vi "Feature extraction.vi"(10 "Utterance Frames":dbl[][](array[numeric])) -> (2 "Acoustic vector":dbl[][](array[numeric]))   [LabVIEW 2013]
uses:
  <vilib>/Analysis/2dsp.llb/Real FFT.vi
  <vilib>/Analysis/2dsp.llb/1D DCT.vi
  <vilib>/Analysis/baseanly.llb/Mean (DBL).vi
  <vilib>/Analysis/NI_AALPro.lvlib
  <vilib>/Analysis/NI_AALBase.lvlib
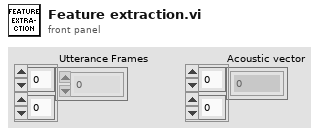
[diagram p1: front panel]
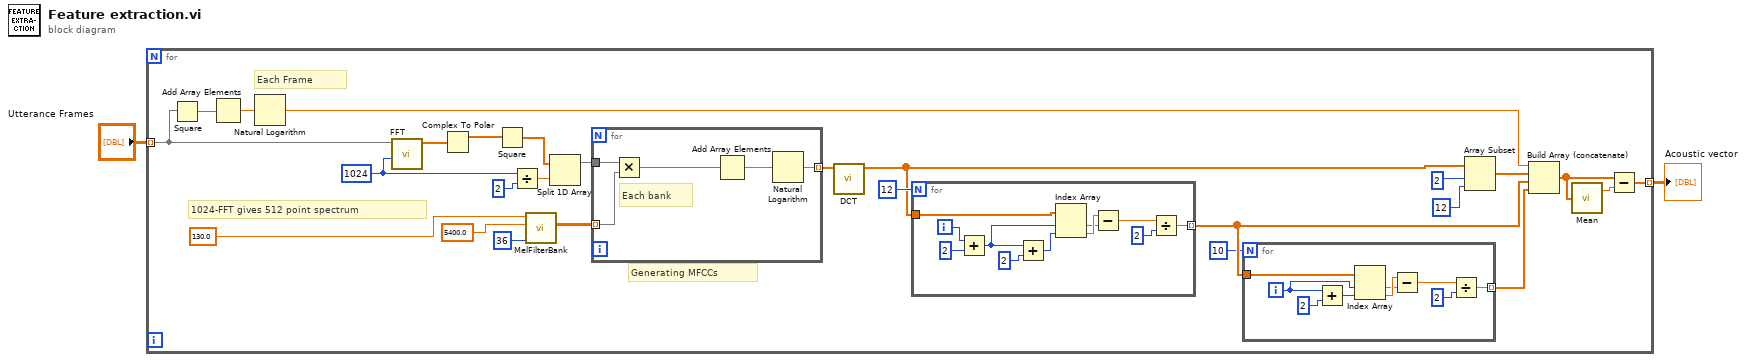
[diagram p0: block diagram]
diagram:
  n1 = for {
    tunnel: "Utterance Frames" -> [w17] mode=indexing
    tunnel: [w3] -> w2 mode=indexing
    w21 = 1024 ("FFT size")
    # "Each Frame"
    # "Generating MFCCs"
    # "1024-FFT gives 512 point spectrum"
    n2 = Square(x=w17) -> (x^2=w16:dbl[])
    n3 = Add Array Elements(numeric array=w16) -> (sum=w15:dbl)
    n4 = Natural Logarithm(1:w15) -> (0:w10:dbl)
    n5 = call-poly <vilib>:"FFT.vi"("FFT size"=w21, "X"=w17) -> ("FFT {X}"=w23:cdb[])  [unwired: 8 in, 1 out]
    n6 = Complex To Polar(r * e^(i*theta)=w23) -> (r=w22:dbl[])  [unwired: 1 out]
    n7 = Square(x=w22) -> (x^2=w18:dbl[])
    n8 = Divide(x=w21, y=2 ("FFT size")) -> (x/y=w19:dbl)
    n9 = call "MelFilterBank.vi"("No of filters"=36, "MaxFreq"=5400.0, "MinFreq"=130.0) -> ("Triangle Pattern"=w25:dbl[][])  [unwired: 6 in]
    n10 = Split 1D Array(array=w18, index=w19) -> (first subarray=w29:dbl[])  [unwired: 1 out]
    n11 = for {
      tunnel: w25 -> [w53] mode=indexing
      tunnel: [w51] -> w24 mode=indexing
      tunnel: w29 -> [w50]
      # "Each bank"
      n12 = Multiply(x=w50, y=w53) -> (x*y=w54:dbl[])
      n13 = Add Array Elements(numeric array=w54) -> (sum=w52:dbl)
      n14 = Natural Logarithm(1:w52) -> (0:w51:dbl)
    }
    n15 = call-poly <vilib>:"DCT.vi"("X"=w24) -> ("DCT {X}"=w13:dbl[])  [unwired: 9 in, 1 out]
    n16 = for {
      N: 12 -> [_]
      tunnel: w13 -> [w49]
      tunnel: [w42] -> w6 mode=indexing
      i -> [w47]
      n17 = Add(x=w47, y=2) -> (x+y=w39:i32)
      n18 = Add(x=w39, y=2) -> (x+y=w40:i32)
      n19 = Index Array(array=w49, index #1=w39, index #2=w40) -> (element #1=w45:dbl, element #2=w46:dbl)
      n20 = Subtract(x=w46, y=w45) -> (x-y=w44:dbl)
      n21 = Divide(x=w44, y=2) -> (x/y=w42:dbl)
    }
    n22 = for {
      N: 10 -> [_]
      tunnel: w6 -> [w38]
      tunnel: [w32] -> w4 mode=indexing
      i -> [w31]
      n23 = Add(x=w31, y=2) -> (x+y=w30:i32)
      n24 = Index Array(array=w38, index #1=w31, index #2=w30) -> (element #1=w35:dbl, element #2=w36:dbl)
      n25 = Subtract(x=w36, y=w35) -> (x-y=w34:dbl)
      n26 = Divide(x=w34, y=2) -> (x/y=w32:dbl)
    }
    n27 = Array Subset(array=w13, index=2, length=12 ("index")) -> (w9:dbl[])
    n28 = Build Array (concatenate)(w10, w9, w6, w4) -> (w7:dbl[])
    n29 = call-poly <vilib>:"Mean.vi"("X"=w7) -> ("mean"=w8:dbl)  [unwired: 1 out]
    n30 = Subtract(x=w7, y=w8) -> (x-y=w3:dbl[])
  }
  "Acoustic vector" <- w2
